vi "通信状态入队列.vi"(8 "错误输入（无错误）":errorcluster, 10 "发送报文":string, 11 "枚举":enum16{"打开连接", "发送数据", "读取数据", "数据处理", "关闭连接"}(ring)) -> (0 "错误输出":errorcluster)   [LabVIEW 2016, in "数据传输系统.lvlib"]
panel:
  out "data":T1
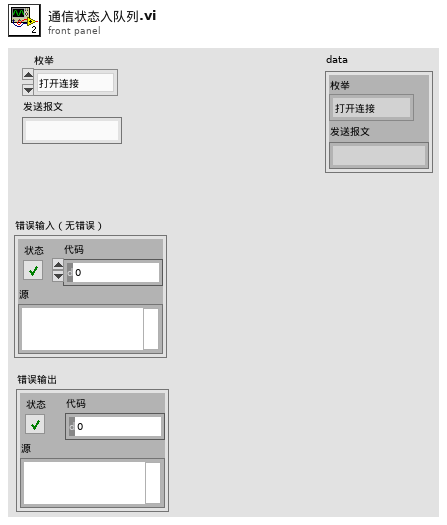
[diagram p1: front panel]
types:
  T1 = cluster{"枚举":enum16{"打开连接", "发送数据", "读取数据", "数据处理", "关闭连接"}, "发送报文":string}
  T2 = cluster{"setini":string, "sysini":string, "hechaini":string, "actualwrite":string, "actualread":string, "datasent":string, "反控命令信息队列":string, "反控与仪器交互":string}
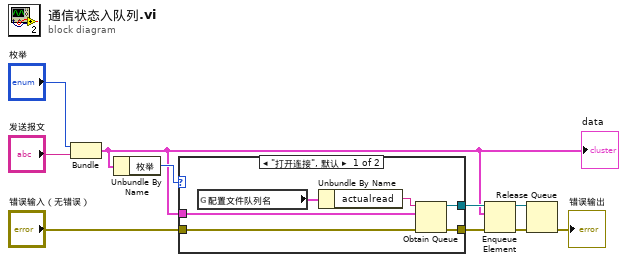
[diagram p0: block diagram]
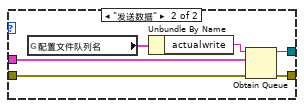
[diagram p2: hidden frame]
diagram:
  n1 = Bundle("枚举"="枚举", "发送报文"="发送报文") -> (w1:T1)  [unwired: 1 in]
  "data" <- w1
  n2 = Unbundle By Name(w1) -> ("枚举"=w4:enum16{"打开连接", "发送数据", "读取数据", "数据处理", "关闭连接"})
  n3 = case shown="\"打开连接\", 默认" w4 {
    tunnel: [w16 w22] -> w9
    tunnel: [w15 w21] -> w8
    tunnel: "错误输入（无错误）" -> [w14 w20]
    tunnel: w1 -> [w11 w17]
    frame "打开连接", Default {
      n4 = global read "断电保存全局.vi" "配置文件队列名"() -> (w13:T2)
      n5 = Unbundle By Name(w13) -> ("actualread"=w12:string)
      n6 = Obtain Queue(name (unnamed)=w12, element data type=w11, error in (no error)=w14) -> (queue out=w16:refnum<queue>, error out=w15:errorcluster)  [unwired: 2 in, 1 out]
    }
    frame "发送数据" {
      n7 = global read "断电保存全局.vi" "配置文件队列名"() -> (w19:T2)
      n8 = Unbundle By Name(w19) -> ("actualwrite"=w18:string)
      n9 = Obtain Queue(name (unnamed)=w18, element data type=w17, error in (no error)=w20) -> (queue out=w22:refnum<queue>, error out=w21:errorcluster)  [unwired: 2 in, 1 out]
    }
  }
  n10 = Enqueue Element(queue=w9, element=w1, error in (no error)=w8) -> (queue out=w10:refnum<queue>, error out=w7:errorcluster)  [unwired: 1 in, 1 out]
  n11 = Release Queue(queue=w10, error in (no error)=w7) -> (error out=→"错误输出":errorcluster)  [unwired: 1 in, 2 out]
